vi "Quick Usb Start Fpga Configuration.vi"(8 "error in (no error)":errorcluster, 11 "hDevice":u32) -> (0 "error out":errorcluster, 2 "function return":i32, 3 "hDevice out":u32)   [LabVIEW 2011, in "QuickUSB.lvlib"]
doc: "QUSBLIB QRETURN QuickUsbStartFpgaConfiguration(\n QHANDLE hDevice\n);"
uses:
  QuickUSB.lvlib
  QuickUSB.dll
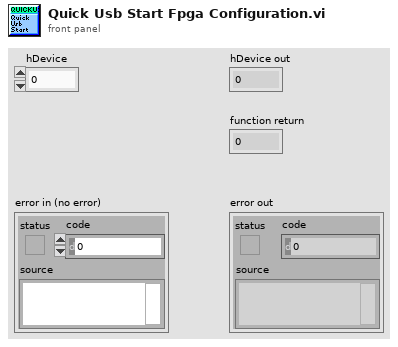
[diagram p1: front panel]
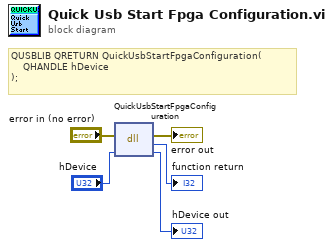
[diagram p0: block diagram]
diagram:
  # "QUSBLIB QRETURN QuickUsbStartFpgaConfiguration(\n    QHANDLE hDevice\n);"
  n1 = dll-call lib="C:/QuickUSB/QuickUSB.*" fn="QuickUsbStartFpgaConfiguration"(error in="error in (no error)", "hDevice"="hDevice") -> (error out=→"error out":errorcluster, →"function return":i32, "hDevice"=→"hDevice out":u32)  [unwired: 2 in, 1 out]
